vi "Main.vi"() -> ()   [LabVIEW 2023]
doc: "This template is for the Queued Message Handler design pattern.\n\nThe Event Handling Loop generates messages based on user interface actions.\n\nThe Message Handling Loop processes messages generated by the Event Handling Loop, or by other messages. The messages are string values, so new messages can be added easily to the Message Cases case structure in the Message Handling Loop. Each message cluster can also provide an optional value for Message Data, which is a variant that can be converted to whatever message-specific data is required."
uses:
  controls/UI Data.ctl
  support/Message Queue/Enqueue Message (Single).vi
  <vilib>/Utility/error.llb/Error Cluster From Error Code.vi
  <vilib>/ErrorRing/Error Ring.xnode
  support/Message Queue/Message Queue.lvlib
  support/User Event - Stop/User Event - Stop.lvlib
panel:
  out "Date&time string":string
  in  "Bulb Switch":bool
  out "Bulb":bool
  out "Display <Replace Me>":string
  in  "Do Something Else <Replace Me>":bool
  in  "Do Something <Replace Me>":bool
  in  "Exit":bool
  # "These controls have associated \"Value Changed\" events configured in the Event Structure on the diagram.\n\nReplace them (and reconfigure the Event Structure) with the controls you need for your application."
  # "This template is for the Queued Message Handler design pattern.\n\nSee the block diagram for more information on how to use this template."
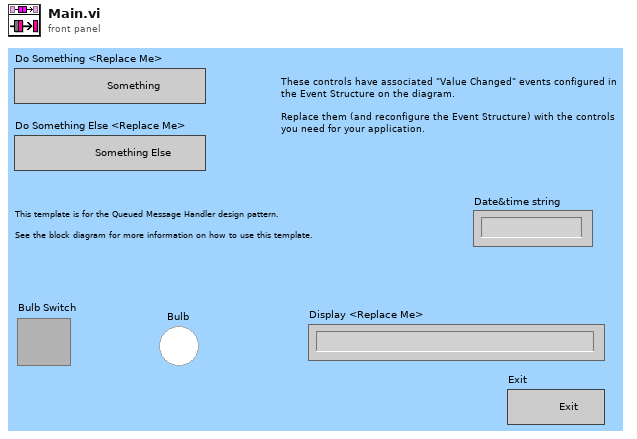
[diagram p1: front panel]
types:
  T1 = typedef "UI Data.ctl" = cluster{"Boolean <Replace Me>":bool, "String <Replace Me>":string, "Numeric <Replace Me>":dbl, "Do Something Ref":refnum<vi>, "Do Something Else Ref":refnum<vi>, "Data Display Ref":refnum<vi>, "Exit Button Ref":refnum<vi>}
  T2 = typedef "Message Queue.lvlib/All Message Queues.ctl" = cluster{"UI":refnum<queue>}
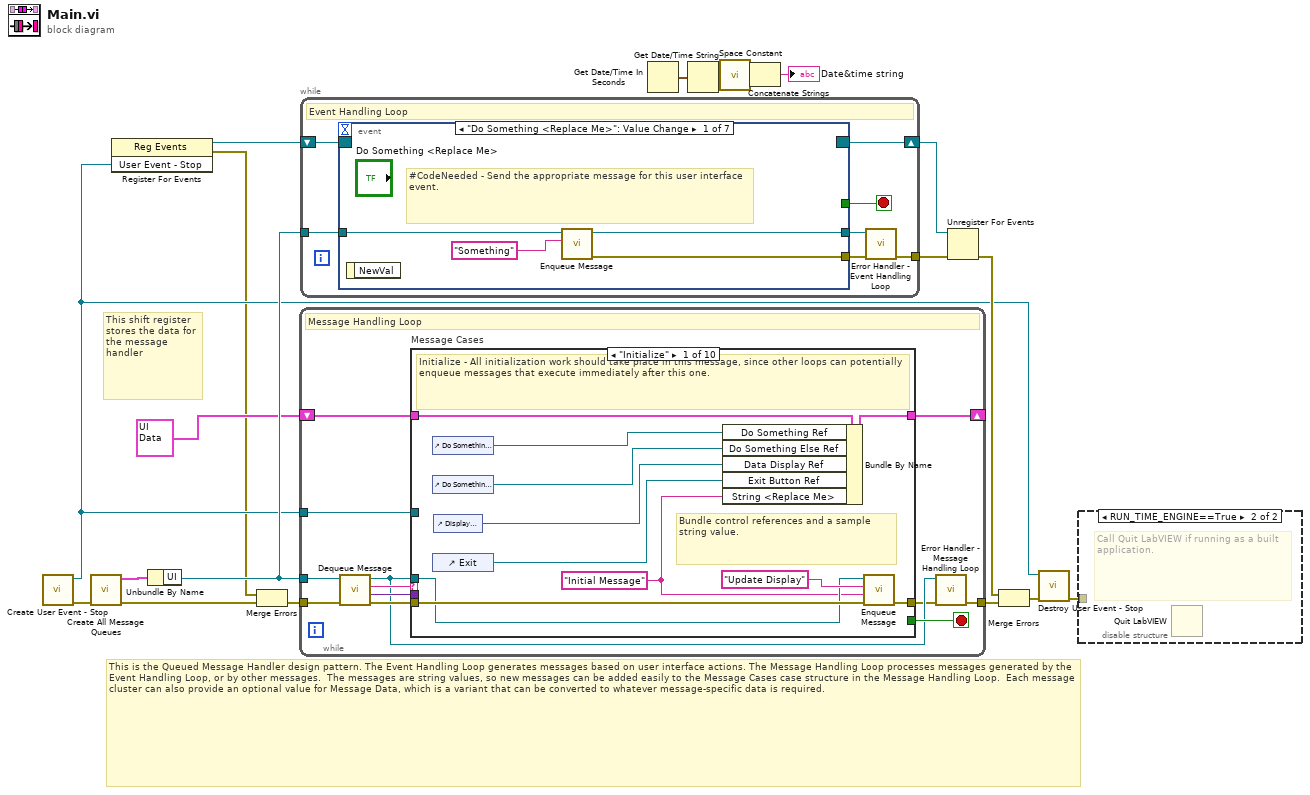
[diagram p0: block diagram]
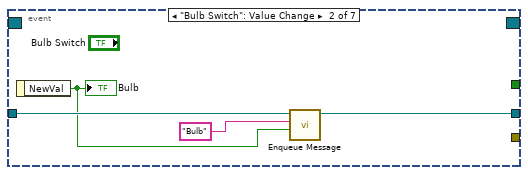
[diagram p3: hidden frame]
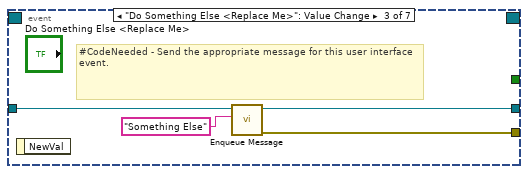
[diagram p4: hidden frame]
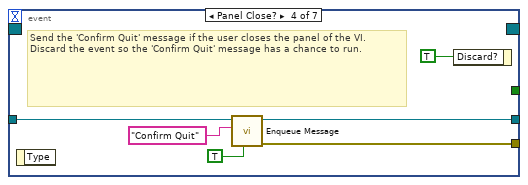
[diagram p5: hidden frame]
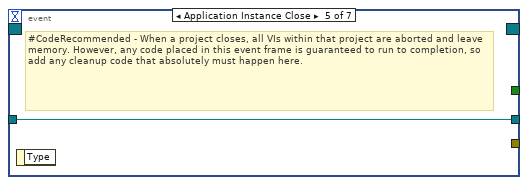
[diagram p6: hidden frame]
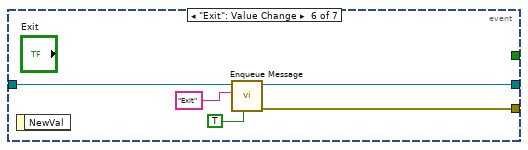
[diagram p7: hidden frame]
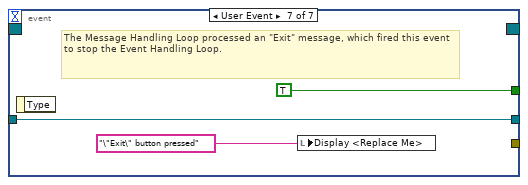
[diagram p8: hidden frame]
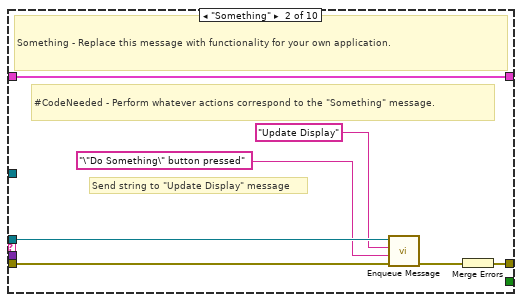
[diagram p9: hidden frame]
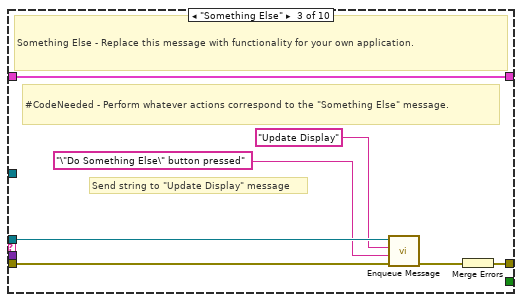
[diagram p10: hidden frame]
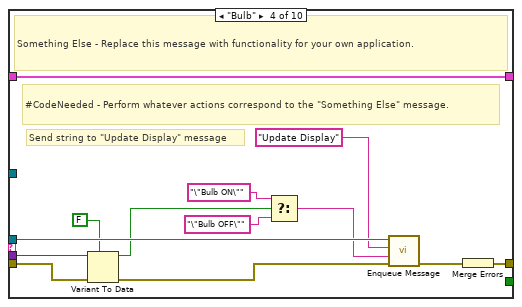
[diagram p11: hidden frame]
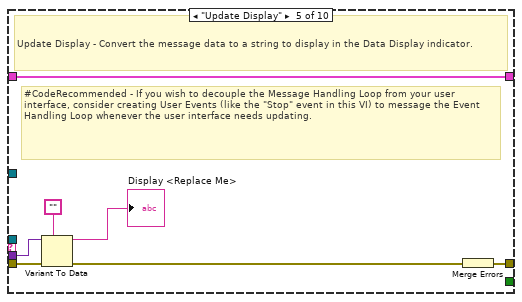
[diagram p12: hidden frame]
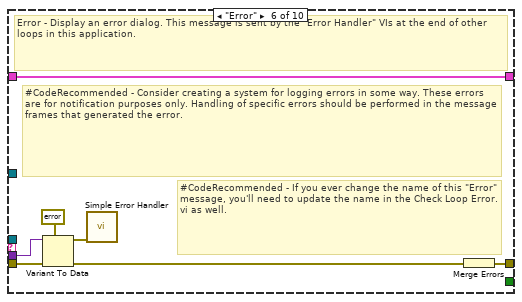
[diagram p13: hidden frame]
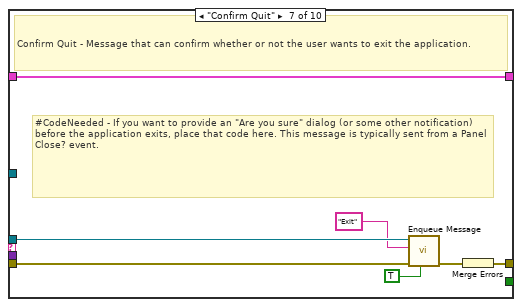
[diagram p14: hidden frame]
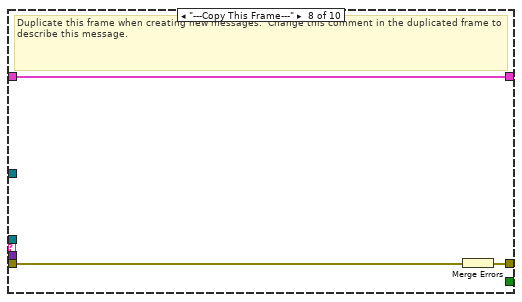
[diagram p15: hidden frame]
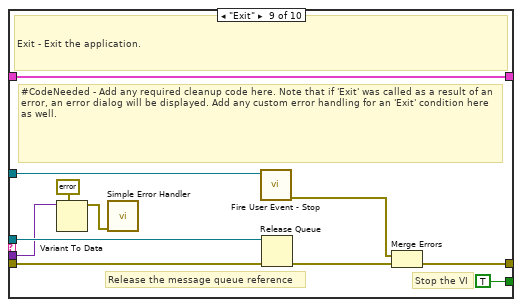
[diagram p16: hidden frame]
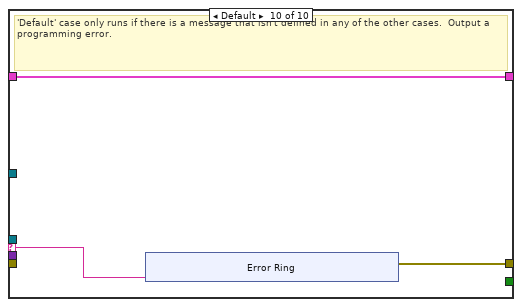
[diagram p17: hidden frame]
diagram:
  # "This is the Queued Message Handler design pattern. The Event Handling Loop generates messages based on user interface actions. The Message Handling Loop processes messages generated by the Event Handling Loop, or by other messages.  The messages are string values, so new messages can be added easily to the Message Cases case structure in the Message Handling Loop.  Each message cluster can also provide an optional value for Message Data, which is a variant that can be converted to whatever message-specific data is required."
  # "This shift register stores the data for the message handler"
  n1 = call "Create User Event - Stop.vi"() -> ("error out"=w16:errorcluster, "User Event - Stop"=w8:refnum<user-event>)  [unwired: 10 in]
  n2 = call "Create All Message Queues.vi"("error in (no error)"=w16) -> ("error out"=w20:errorcluster, "Message Queues out"=w19:T2)  [unwired: 9 in]
  n3 = register-events(w8) -> (reference out=w9:refnum<event-registration>, error out=w6:errorcluster)  [unwired: 2 in]
  n4 = Unbundle By Name(w19) -> ("UI"=w17:refnum<queue>)
  n5 = Merge Errors(w6, w20) -> (w7:errorcluster)
  n6 = while {
    tunnel: w17 -> [w24]
    shift-right: [w31] -> _
    shift-left: T1 {"Boolean <Replace Me>"=FALSE, "String <Replace Me>"="", "Numeric <Replace Me>"=0.0, "Do Something Ref"=refnum, "Do Something Else Ref"=refnum, "Data Display Ref"=refnum, "Exit Button Ref"=refnum} ("Data Cluster") -> [w32]
    tunnel: w8 -> [w29]
    tunnel: w7 -> [w28]
    tunnel: [w22] -> w18
    stop <- w30 stop-if-true
    # "Message Handling Loop"
    n7 = call "Dequeue Message.vi"("error in (no error)"=w28, "Message Queue"=w24) -> ("error out"=w27:errorcluster, "Message Data"=w25:variant, "Message"=w26:string, "dup Message Queue"=w23:refnum<queue>)  [unwired: 6 in]
    n8 = case "Message Cases" shown="\"Initialize\"" w26 {
      selector: w26 -> [_ _ _ _ _ _ _ _ _ w106]
      tunnel: w23 -> [w34 w46 w53 w67 _ _ w87 _ w105 _]
      tunnel: w27 -> [w42 w48 w55 w65 w75 w84 w91 w94 w98 _]
      tunnel: [w43 w49 w56 w69 w76 w78 w89 w92 w101 w107] -> w21
      tunnel: w32 -> [w41 w50 w57 w70 w77 w83 w90 w93 w104 w108]
      tunnel: [w40 w50 w57 w70 w77 w83 w90 w93 w104 w108] -> w31
      tunnel: [_ _ _ _ _ _ _ _ TRUE _] -> w30
      tunnel: w25 -> [_ _ _ w63 w74 w82 _ _ w95 _]
      tunnel: w29 -> [_ _ _ _ _ _ _ _ w100 _]
      frame "Initialize" {
        w33 = "Initial Message" ("Initial Message")
        # "Bundle control references and a sample string value."
        # "Initialize - All initialization work should take place in this message, since other loops can potentially enqueue messages that execute immediately after this one."
        n9 = control-ref of="Do Something <Replace Me>"() -> (w39:refnum<vi>)
        n10 = control-ref of="Do Something Else <Replace Me>"() -> (w38:refnum<vi>)
        n11 = control-ref of="Exit"() -> (w36:refnum<vi>)
        n12 = control-ref of="Display <Replace Me>"() -> (w37:refnum<vi>)
        n13 = Bundle By Name(cluster=w41, "Do Something Ref"=w39, "Do Something Else Ref"=w38, "Data Display Ref"=w37, "Exit Button Ref"=w36, "String <Replace Me>"=w33) -> (w40:T1)
        n14 = call-poly "Enqueue Message.vi"("error in (no error)"=w42, "Message Data"=w33, "Message"="Update Display", "Message Queue"=w34) -> ("error out"=w43:errorcluster)  [unwired: 6 in, 1 out]
      }
      frame "Something" {
        # "Send string to \"Update Display\" message"
        # "#CodeNeeded - Perform whatever actions correspond to the \"Something\" message."
        # "Something - Replace this message with functionality for your own application."
        n15 = call-poly "Enqueue Message.vi"("error in (no error)"=w48, "Message Data"="\"Do Something\" button pressed" ("\"Do Something\" button pressed"), "Message"="Update Display", "Message Queue"=w46) -> ("error out"=w47:errorcluster)  [unwired: 6 in, 1 out]
        n16 = Merge Errors(w47) -> (w49:errorcluster)
      }
      frame "Something Else" {
        # "Send string to \"Update Display\" message"
        # "#CodeNeeded - Perform whatever actions correspond to the \"Something Else\" message."
        # "Something Else - Replace this message with functionality for your own application."
        n17 = call-poly "Enqueue Message.vi"("error in (no error)"=w55, "Message Data"="\"Do Something Else\" button pressed" ("\"Do Something Else\" button pressed"), "Message"="Update Display", "Message Queue"=w53) -> ("error out"=w54:errorcluster)  [unwired: 6 in, 1 out]
        n18 = Merge Errors(w54) -> (w56:errorcluster)
      }
      frame "Bulb" {
        # "Send string to \"Update Display\" message"
        # "#CodeNeeded - Perform whatever actions correspond to the \"Something Else\" message."
        # "Something Else - Replace this message with functionality for your own application."
        n19 = Variant To Data(error in=w65, type=FALSE, Variant=w63) -> (data=w61:bool, error out=w64:errorcluster)
        n20 = Select(t="\"Bulb ON\"" ("\"Do Something Else\" button pressed"), s=w61, f="\"Bulb OFF\"" ("\"Do Something Else\" button pressed")) -> (s? t:f=w59:string)
        n21 = call-poly "Enqueue Message.vi"("error in (no error)"=w64, "Message Data"=w59, "Message"="Update Display", "Message Queue"=w67) -> ("error out"=w68:errorcluster)  [unwired: 6 in, 1 out]
        n22 = Merge Errors(w68) -> (w69:errorcluster)
      }
      frame "Update Display" {
        # "#CodeRecommended - If you wish to decouple the Message Handling Loop from your user interface, consider creating User Events (like the \"Stop\" event in this VI) to message the Event Handling Loop whenever the user interface needs updating."
        # "Update Display - Convert the message data to a string to display in the Data Display indicator."
        n23 = Variant To Data(error in=w75, type="", Variant=w74) -> (data=→"Display <Replace Me>":string, error out=w72:errorcluster)
        n24 = Merge Errors(w72) -> (w76:errorcluster)
      }
      frame "Error" {
        # "#CodeRecommended - If you ever change the name of this \"Error\" message, you'll need to update the name in the Check Loop Error.vi as well."
        # "#CodeRecommended - Consider creating a system for logging errors in some way. These errors are for notification purposes only. Handling of specific errors should be performed in the message frames that generated the error."
        # "Error - Display an error dialog. This message is sent by the \"Error Handler\" VIs at the end of other loops in this application."
        n25 = Variant To Data(error in=w84, type=errorcluster {"status"=FALSE, "code"=0, "source"=""} ("error constant"), Variant=w82) -> (data=w80:errorcluster, error out=w79:errorcluster)
        n26 = call <vilib>:"Simple Error Handler.vi"("error in (no error)"=w80) -> ()  [unwired: 4 in, 5 out]
        n27 = Merge Errors(w79) -> (w78:errorcluster)
      }
      frame "Confirm Quit" {
        # "#CodeNeeded - If you want to provide an \"Are you sure\" dialog (or some other notification) before the application exits, place that code here. This message is typically sent from a Panel Close? event."
        # "Confirm Quit - Message that can confirm whether or not the user wants to exit the application."
        n28 = call-poly "Enqueue Message.vi"("Priority Message? (F)"=TRUE, "error in (no error)"=w91, "Message"="Exit", "Message Queue"=w87) -> ("error out"=w88:errorcluster)  [unwired: 6 in, 1 out]
        n29 = Merge Errors(w88) -> (w89:errorcluster)
      }
      frame "---Copy This Frame---" {
        # "Duplicate this frame when creating new messages.  Change this comment in the duplicated frame to describe this message."
        n30 = Merge Errors(w94) -> (w92:errorcluster)
      }
      frame "Exit" {
        # "Stop the VI"
        # "Release the message queue reference"
        # "#CodeNeeded - Add any required cleanup code here. Note that if 'Exit' was called as a result of an error, an error dialog will be displayed. Add any custom error handling for an 'Exit' condition here as well."
        # "Exit - Exit the application."
        n31 = Variant To Data(type=errorcluster {"status"=FALSE, "code"=0, "source"=""} ("error constant"), Variant=w95) -> (data=w96:errorcluster)  [unwired: 1 in, 1 out]
        n32 = call <vilib>:"Simple Error Handler.vi"("error in (no error)"=w96) -> ()  [unwired: 4 in, 5 out]
        n33 = call "Fire User Event - Stop.vi"("User Event - Stop"=w100) -> ("error out"=w99:errorcluster)  [unwired: 10 in]
        n34 = Release Queue(queue=w105, error in (no error)=w98) -> (error out=w102:errorcluster)  [unwired: 1 in, 2 out]
        n35 = Merge Errors(w99, w102) -> (w101:errorcluster)
      }
      frame Default {
        # "'Default' case only runs if there is a message that isn't defined in any of the other cases.  Output a programming error."
        n36 = xnode "Error Ring"("parameter 0"=w106) -> ("error out"=w107:errorcluster)
      }
    }
    n37 = call "Error Handler - Message Handling Loop.vi"("error in (no error)"=w21, "Message Queue"=w23) -> ("dup error in"=w22:errorcluster)  [unwired: 8 in, 1 out]
  }
  n38 = while {
    tunnel: w17 -> [w122]
    shift-right: [w120] -> w13
    shift-left: w9 -> [w121]
    tunnel: [w116] -> w10
    stop <- w118 stop-if-true
    # "Event Handling Loop"
    n39 = event shown="[0] \"Do Something <Replace Me>\": Value Change" {
      selector: w121 -> [_ _ _ _ _ _ _]
      dyn-events: [_ _ _ _ _ _ _] -> w120
      timeout: _ -> [_ _ _ _ _ _ _]
      tunnel: [_ _ _ _ _ _ TRUE ("Discard?")] -> w118
      tunnel: w122 -> [w126 w130 w134 w139 w141 w146 w149]
      tunnel: [w123 _ w131 w138 _ w145 _] -> w119
      tunnel: [w125 w129 w133 w137 w141 w144 w149] -> w117
      event "Do Something <Replace Me>": Value Change {
        # "#CodeNeeded - Send the appropriate message for this user interface event."
        n40 = event-data() -> ()  [unwired: 1 in, 1 out]
        n41 = call-poly "Enqueue Message.vi"("Message"="Something", "Message Queue"=w126) -> ("error out"=w123:errorcluster, "dup Message Queue"=w125:refnum<queue>)  [unwired: 8 in]
      }
      event "Bulb Switch": Value Change {
        n42 = event-data() -> ("NewVal"=w127:bool)  [unwired: 1 in]
        "Bulb" <- w127
        n43 = call-poly "Enqueue Message.vi"("Message Data"=w127, "Message"="Bulb", "Message Queue"=w130) -> ("dup Message Queue"=w129:refnum<queue>)  [unwired: 7 in, 1 out]
      }
      event "Do Something Else <Replace Me>": Value Change {
        # "#CodeNeeded - Send the appropriate message for this user interface event."
        n44 = event-data() -> ()  [unwired: 1 in, 1 out]
        n45 = call-poly "Enqueue Message.vi"("Message"="Something Else", "Message Queue"=w134) -> ("error out"=w131:errorcluster, "dup Message Queue"=w133:refnum<queue>)  [unwired: 8 in]
      }
      event Panel Close? {
        # "Send the 'Confirm Quit' message if the user closes the panel of the VI. Discard the event so the 'Confirm Quit' message has a chance to run."
        n46 = event-data() -> ()  [unwired: 1 in, 1 out]
        n47 = call-poly "Enqueue Message.vi"("Priority Message? (F)"=TRUE, "Message"="Confirm Quit", "Message Queue"=w139) -> ("error out"=w138:errorcluster, "dup Message Queue"=w137:refnum<queue>)  [unwired: 7 in]
        n48 = event-data("Discard?"=TRUE) -> ()  [unwired: 1 in, 1 out]
      }
      event Application Instance Close {
        # "#CodeRecommended - When a project closes, all VIs within that project are aborted and leave memory. However, any code placed in this event frame is guaranteed to run to completion, so add any cleanup code that absolutely must happen here."
        n49 = event-data() -> ()  [unwired: 1 in, 1 out]
      }
      event "Exit": Value Change {
        n50 = event-data() -> ()  [unwired: 1 in, 1 out]
        n51 = call-poly "Enqueue Message.vi"("Priority Message? (F)"=TRUE, "Message"="Exit", "Message Queue"=w146) -> ("error out"=w145:errorcluster, "dup Message Queue"=w144:refnum<queue>)  [unwired: 7 in]
      }
      event User Event {
        # "The Message Handling Loop processed an \"Exit\" message, which fired this event to stop the Event Handling Loop."
        n52 = event-data() -> ()  [unwired: 1 in, 1 out]
        n53 = local write "Display <Replace Me>"("\"Exit\" button pressed" ("VI Stopped")) -> ()
      }
    }
    n54 = call "Error Handler - Event Handling Loop.vi"("error in (no error)"=w119, "Message Queue"=w117) -> ("dup error in"=w116:errorcluster)  [unwired: 8 in, 1 out]
  }
  n55 = Get Date/Time In Seconds() -> (seconds since 1Jan1904=w5:timestamp)
  n56 = Get Date/Time String(seconds (now)=w5) -> (date string=w4:string, time string=w2:string)  [unwired: 2 in]
  n57 = call <vilib>:"Space Constant.vi"() -> ("String"=w1:string)
  n58 = Concatenate Strings(w4, w1, w2) -> (→"Date&time string":string)
  n59 = Unregister For Events(event registration refnum=w13, error in=w10) -> (error out=w14:errorcluster)
  n60 = Merge Errors(w14, w18) -> (w15:errorcluster)
  n61 = call "Destroy User Event - Stop.vi"("error in (no error)"=w15, "User Event - Stop"=w8) -> ("error out"=w11:errorcluster)  [unwired: 9 in]
  n62 = disable-structure shown="RUN_TIME_ENGINE==True" {
    disable-tunnel: w11 -> [_ _]
    frame condition #0 (active) {
    }
    frame condition #1 {
      # "Call Quit LabVIEW if running as a built application."
      n63 = Quit LabVIEW() -> ()  [unwired: 1 in]
    }
  }
